vi "Get Variable List String.vi"(8 "error in (no error)":errorcluster, 10 "Variable Type":enum16{"Project", "Execution"}(ring), 11 "Project in":refnum<class "Project.lvclass">) -> (0 "error out":errorcluster, 2 "Names":string, 3 "Project out":refnum<class "Project.lvclass">)   [LabVIEW 2015, in "Project.lvclass"]
uses:
  Project.lvclass
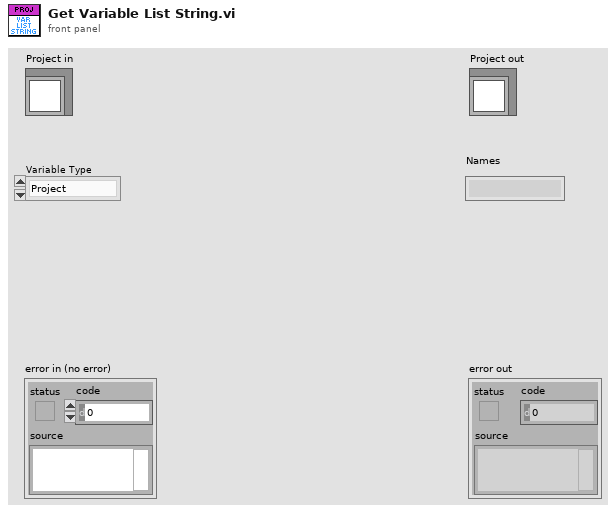
[diagram p1: front panel]
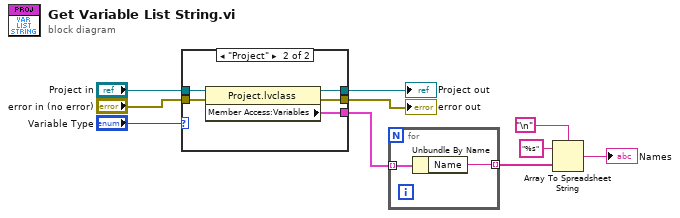
[diagram p0: block diagram]
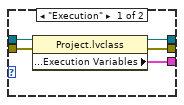
[diagram p2: hidden frame]
diagram:
  n1 = case shown="\"Project\"" "Variable Type" {
    tunnel: "Project in" -> [w15 w20]
    tunnel: "error in (no error)" -> [w14 w19]
    tunnel: [w13 w18] -> w7
    tunnel: [w12 w17] -> w6
    tunnel: [w11 w16] -> w5
    frame "Execution" {
      n2 = property class="Project.lvclass"(reference=w15, error in=w14) -> (reference out=w13:refnum<class "Project.lvclass">, error out=w12:errorcluster, "Member Access:Execution Variables"=w11:cluster{"Name":string, "Value":variant}[])
    }
    frame "Project" {
      n3 = property class="Project.lvclass"(reference=w20, error in=w19) -> (reference out=w18:refnum<class "Project.lvclass">, error out=w17:errorcluster, "Member Access:Variables"=w16:cluster{"Name":string, "Value":variant}[])
    }
  }
  "error out" <- w6
  "Project out" <- w7
  n4 = for {
    tunnel: w5 -> [w22] mode=indexing
    tunnel: [w21] -> w2 mode=indexing
    n5 = Unbundle By Name(w22) -> ("Name"=w21:string)
  }
  n6 = Array To Spreadsheet String(delimiter (Tab)="\n", array=w2, 3:"%s" ("format string")) -> (spreadsheet string=→"Names":string)
